vi "Msg.vi"(7 "Actor in":refnum<class "Actor.lvclass">, 11 "Destroy Self Msg in":refnum<class "Destroy Self Msg.lvclass">) -> (0 "Error out":errorcluster, 5 "Actor out":refnum<class "Actor.lvclass">)   [LabVIEW 2025, in "jettl.lvlib" / "Destroy Self Msg.lvlib" / "Destroy Self Msg.lvclass"]
uses:
  Destroy Self Msg.lvclass
  Destroy Self Msg.lvclass/Destroy Self Msg.ctl
  Destroy Self/Destroy Self.lvclass
  Actor/Actor/Actor.lvclass
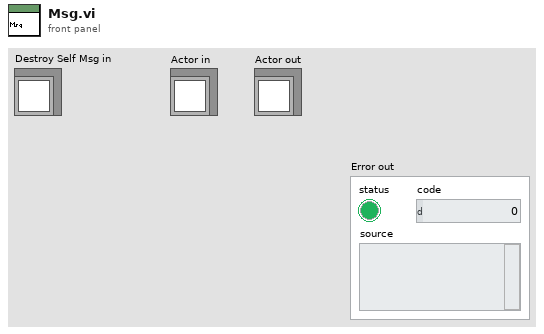
[diagram p1: front panel]
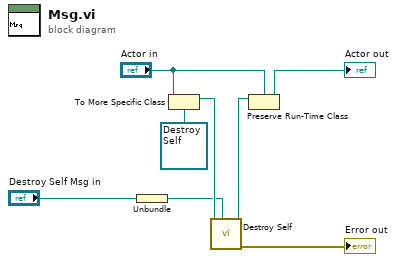
[diagram p0: block diagram]
diagram:
  n1 = Unbundle "Unbundle"("Destroy Self Msg in") -> (w2:refnum<class "Sender.lvclass">)
  n2 = To More Specific Class(target class=refnum<class "Destroy Self.lvclass"> refnum ("Destroy.lvlib:Destroy.lvclass"), reference="Actor in") -> (specific class reference=w4:refnum<class "Destroy Self.lvclass">)  [unwired: 1 in, 1 out]
  n3 = call-dynamic "Destroy Self.vi"("Sender"=w2, "Destroy Self in"=w4) -> ("Error out"=→"Error out":errorcluster, "Destroy Self out"=w3:refnum<class "Destroy Self.lvclass">)  [unwired: 8 in]
  n4 = Preserve Run-Time Class(object in=w3, 2:"Actor in") -> (object out=→"Actor out":refnum<class "Actor.lvclass">)  [unwired: 1 in, 1 out]
